vi "ACQ read summary file.vi"(10 "ACQ binary data file path":path) -> (0 "Total of events":string, 1 "ID summary":string, 2 "quants events per chip":u32[](array[numeric]), 3 "ChipID list":u32[](array[numeric]) format="%.0x")   [LabVIEW 2015, in "VIPM2.lvlib"]
doc: "Llegeix el ACQ summary file i construeix les variables per al Data viewer."
uses:
  VIPM2.lvlib
panel:
  out "Chip data text":string
  out "text from file":string
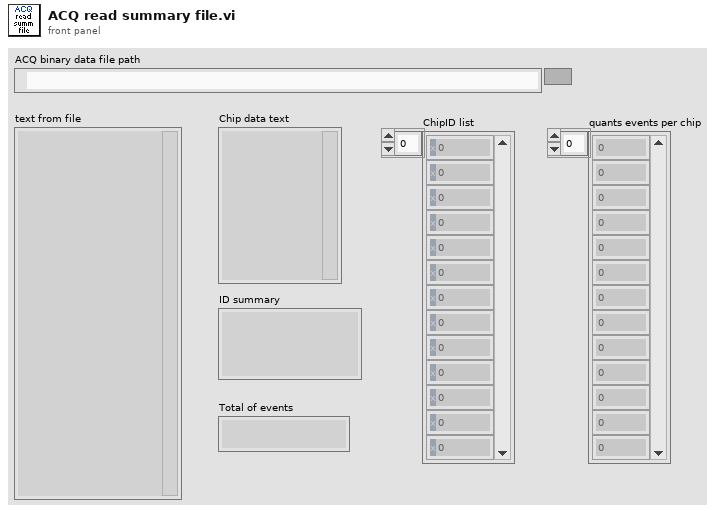
[diagram p1: front panel]
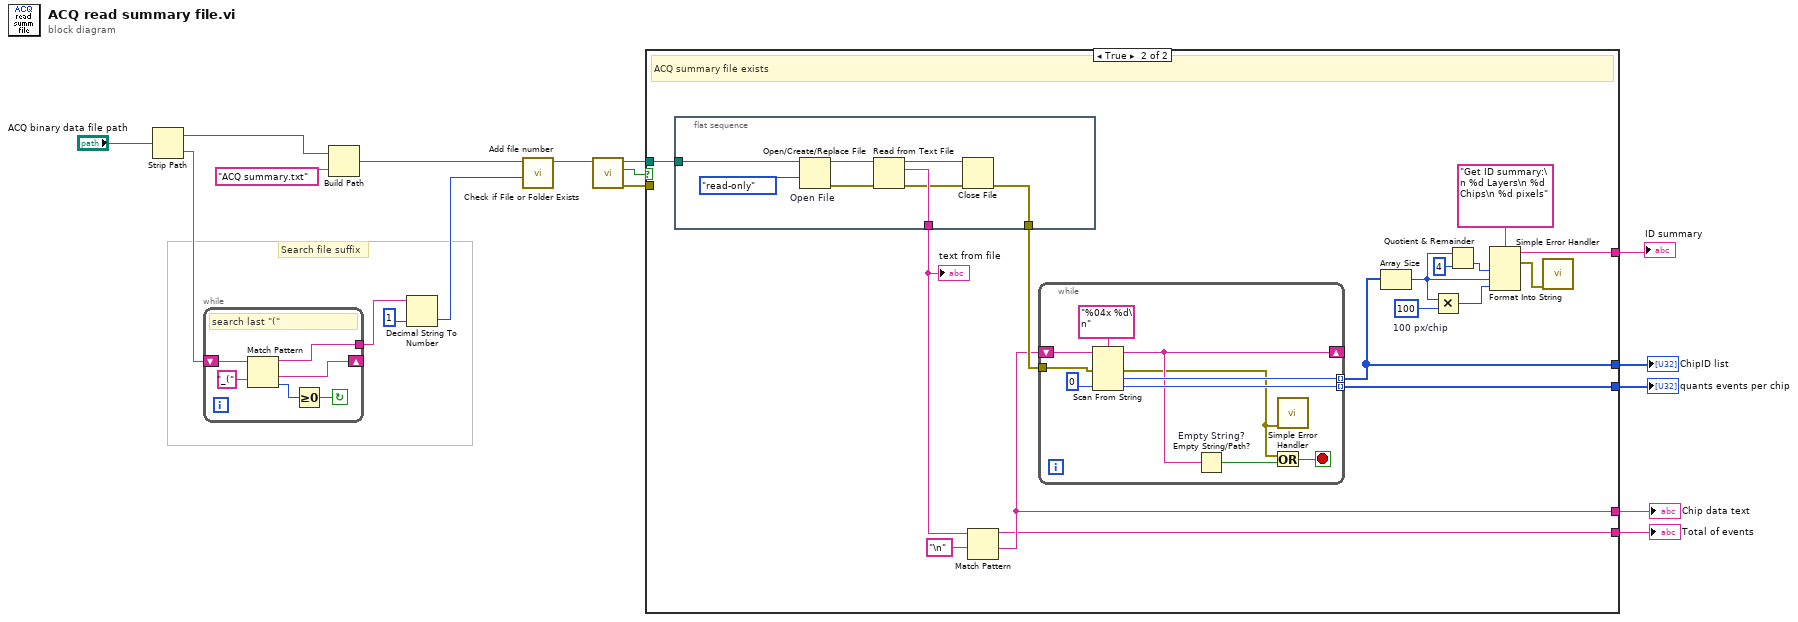
[diagram p0: block diagram]
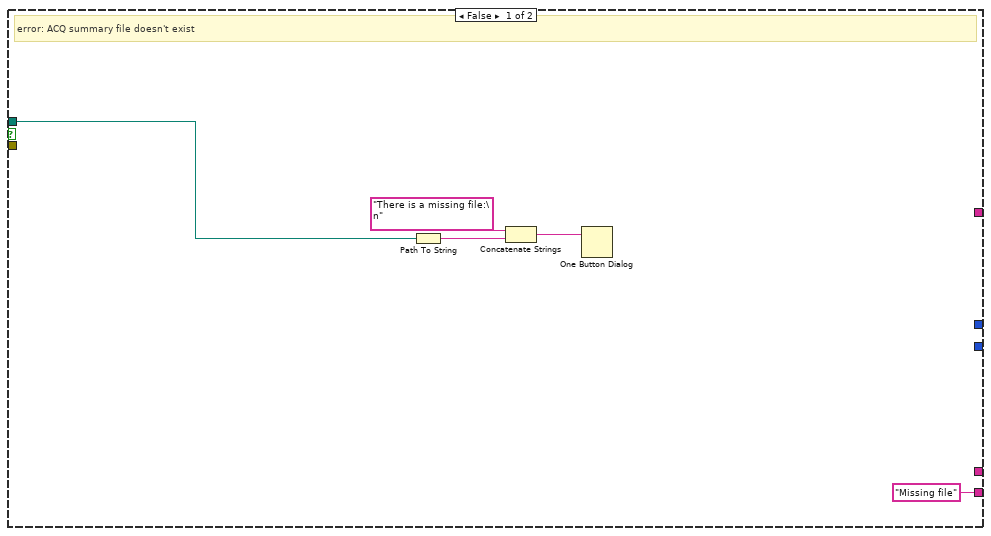
[diagram p2: hidden frame]
diagram:
  # "Search file suffix"
  n1 = Strip Path(path="ACQ binary data file path") -> (stripped path=w12:path, name=w2:string)
  n2 = while {
    shift-right: [w21] -> _
    shift-left: w2 -> [w23]
    tunnel: [w18] -> w4
    stop <- w19 continue-if-true
    # "search last \"(\""
    n3 = Match Pattern(string=w23, regular expression="_(") -> (before substring=w18:string, after substring=w21:string, offset past match=w20:i32)  [unwired: 1 in, 1 out]
    n4 = Greater Or Equal To 0?(x=w20) -> (x >= 0?=w19:bool)
  }
  n5 = Build Path(base path=w12, name or relative path="ACQ summary.txt") -> (appended path=w5:path)
  n6 = Decimal String To Number(string=w4, default (0L)=u32 1 ("default (0 I32)")) -> (number=w1:u32)  [unwired: 1 in, 1 out]
  n7 = call "Add file number.vi"("sufix number"=w1, "file path"=w5) -> ("incremented file path"=w6:path)  [unwired: 9 in]
  n8 = call <vilib>:"Check if File or Folder Exists.vi"("path"=w6) -> ("error out"=w7:errorcluster, "file or folder exists?"=w8:bool, "dup path"=w9:path)  [unwired: 8 in]
  n9 = case shown="True" w8 {
    tunnel: [_ w43] -> w17
    tunnel: [_ w41] -> w16
    tunnel: [_ w35] -> w15
    tunnel: [_ w32] -> w11
    tunnel: ["Missing file" w31] -> w10
    tunnel: w9 -> [w25 w29]
    tunnel: w7 -> [_ _]
    frame False {
      # "error: ACQ summary file doesn't exist"
      n10 = Path To String(path=w25) -> (string=w26:string)
      n11 = Concatenate Strings("There is a missing file:\n" ("string"), w26) -> (w24:string)
      n12 = One Button Dialog(message=w24) -> ()  [unwired: 1 in, 1 out]
    }
    frame True {
      w37 = 100  # 100 px/chip
      # "ACQ summary file exists"
      n13 = flat-sequence {
        tunnel: [w51] -> w44
        tunnel: [w46] -> w33
        tunnel: w29 -> [w45]
        frame #0 {
          n14 = Open/Create/Replace File "Open File"(file path (use dialog)=w45, access (0:read/write)=enum16{"read/write", "read-only", "write-only"}."read-only") -> (refnum out=w50:refnum<file>, error out=w49:errorcluster)  [unwired: 4 in, 1 out]
          n15 = Read from Text File(file (use dialog)=w50, error in=w49) -> (refnum out=w48:refnum<file>, text=w51:string, error out=w47:errorcluster)  [unwired: 2 in, 1 out]
          n16 = Close File(refnum=w48, error in=w47) -> (error out=w46:errorcluster)  [unwired: 1 out]
        }
      }
      n17 = Match Pattern(string=w44, regular expression="\n") -> (before substring=w31:string, after substring=w32:string)  [unwired: 1 in, 2 out]
      n18 = while {
        shift-right: [w55] -> _
        shift-left: w32 -> [w56]
        tunnel: [w58] -> w41 mode=indexing
        tunnel: [w57] -> w43 mode=indexing
        tunnel: w33 -> [w53]
        stop <- w62 stop-if-true
        n19 = Scan From String "Scan From String"(format string="%04x %d\n", input string=w56, error in=w53, default 2=u32 0 ("default value 2")) -> (remaining string=w55:string, error out=w54:errorcluster, output 1=w58:u32, output 2=w57:u32)  [unwired: 2 in, 1 out]
        n20 = Empty String/Path? "Empty String?"(string/path=w55) -> (empty?=w61:bool)
        n21 = Or(x=w54, y=w61) -> (x .or. y?=w62:bool)
        n22 = call <vilib>:"Simple Error Handler.vi"("error in (no error)"=w54) -> ()  [unwired: 4 in, 5 out]
      }
      n23 = Array Size(array=w41) -> (size(s)=w38:i32)
      n24 = Multiply(x=w38, y=w37) -> (x*y=w36:i32)
      n25 = Quotient & Remainder(x=w38, y=4) -> (floor(x/y)=w40:i32)  [unwired: 1 out]
      n26 = Format Into String "Format Into String"(format string="Get ID summary:\n %d Layers\n %d Chips\n %d pixels", w40, w38, w36) -> (resulting string=w35:string, error out=w34:errorcluster)  [unwired: 2 in]
      n27 = call <vilib>:"Simple Error Handler.vi"("error in (no error)"=w34) -> ()  [unwired: 4 in, 5 out]
      "text from file" <- w44
    }
  }
  "Chip data text" <- w11
  "ChipID list" <- w16
  "quants events per chip" <- w17
  "ID summary" <- w15
  "Total of events" <- w10
